vi "get_number_of_consecutive_scan_pixels.vi"(8 "error in (no error)":errorcluster, 11 "GenericTrajectory in":refnum<class "GenericTrajectory.lvclass">) -> (0 "error out":errorcluster, 2 "number of consecutive scan pixels":i64, 3 "GenericTrajectory out":refnum<class "GenericTrajectory.lvclass">)   [LabVIEW 2010, in "GenericTrajectory.lvclass"]
doc: "returns the number of pixels scanned in one piece when in single-sweep mode or experiment mode"
uses:
  GenericTrajectory.lvclass
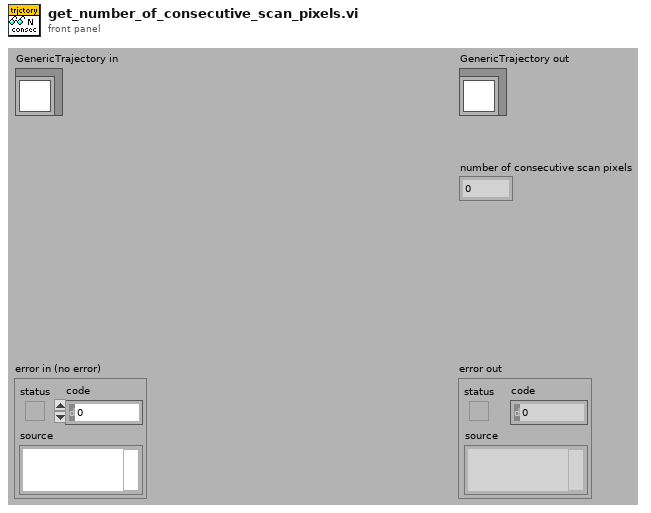
[diagram p1: front panel]
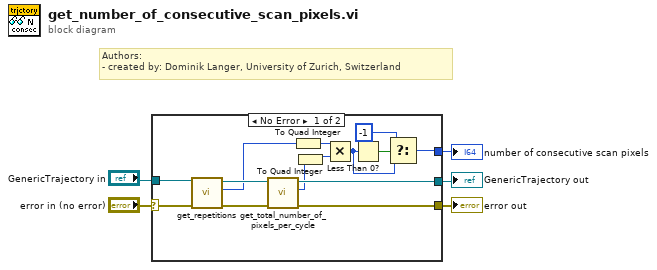
[diagram p0: block diagram]
diagram:
  # "Authors: \n- created by: Dominik Langer, University of Zurich, Switzerland"
  n1 = case shown="No Error" "error in (no error)" {
    selector: "error in (no error)" -> [w17 w21]
    tunnel: [w16 w21] -> w3
    tunnel: [w15 w20] -> w4
    tunnel: "GenericTrajectory in" -> [w18 w20]
    tunnel: [w8 _] -> w5
    frame No Error {
      n2 = call-dynamic "get_repetitions.vi"("error in (no error)"=w17, "GenericTrajectory in"=w18) -> ("error out"=w14:errorcluster, "repetitions"=w10:i32, "GenericTrajectory out"=w19:refnum<class "GenericTrajectory.lvclass">)  [unwired: 7 out]
      n3 = call-dynamic "get_total_number_of_pixels_per_cycle.vi"("error in (no error)"=w14, "GenericTrajectory in"=w19) -> ("error out"=w16:errorcluster, "total number of pixels per cycle"=w12:i32, "GenericTrajectory out"=w15:refnum<class "GenericTrajectory.lvclass">)  [unwired: 7 out]
      n4 = To Quad Integer(1:w10) -> (0:w11:i64)
      n5 = To Quad Integer(1:w12) -> (0:w13:i64)
      n6 = Multiply(x=w11, y=w13) -> (x*y=w7:i64)
      n7 = Less Than 0?(x=w7) -> (x < 0?=w9:bool)
      n8 = Select(t=i64 -1, s=w9, f=w7) -> (s? t:f=w8:i64)
    }
    frame Error {
    }
  }
  "error out" <- w3
  "GenericTrajectory out" <- w4
  "number of consecutive scan pixels" <- w5
